vi "Add Subscriber.vi"(8 "error in (no error)":errorcluster, 10 "New FIFO Instance Config":T1, 11 "CIF_Fifo_Raw_Multi in":refnum<class "CIF_NIChn_Raw.lvclass">) -> (0 "error out":errorcluster, 2 "New Publisher":string, 3 "CIF_Fifo_Raw_Multi out":refnum<class "CIF_NIChn_Raw.lvclass">)   [LabVIEW 2021, in "CIF_NIChn_Raw.lvclass"]
uses:
  CIF_NIChn_Raw.lvclass
  D:/dev/Packages/Channel_Manager/src/CIFChannels/CIFChannels.lvclass
  D:/dev/Packages/Channel_Manager/src/CIF_NIChn/FIFO_U8_Multi/CIF_Fifo_U8_Multi.lvclass
  ChannelCommon/typedef/New FIFO Instance Configuration.ctl
  CIF_NIChn_Raw.lvclass/CIF_NIChn_Raw.ctl
  FIFO_U8_Multi/CIF_Fifo_U8_Multi.lvclass/CIF_Fifo_U8_Multi.ctl
  CIFChannels/Typedef/Direction.ctl
  FIFO_U8_Multi/Accessors/Read Publishers.vi
  FIFO_U8_Multi/Accessors/Write Publishers.vi
  FIFO_U8/CIF_NIChn_Fifo_U8.lvclass
  CIFChannels/CIFChannels.lvclass
  ChannelCommon/ChannelCommon.lvlib
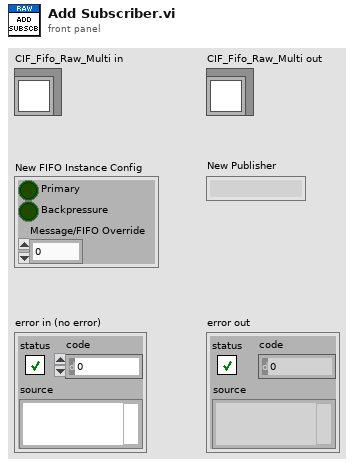
[diagram p1: front panel]
types:
  T1 = typedef "ChannelCommon.lvlib/New FIFO Instance Configuration.ctl" = cluster{"Primary":bool, "Backpressure":bool, "Message/FIFO Override":u32}
  T2 = typedef "CIFChannels.lvclass/Direction.ctl" = enum16{"Publisher", "Subscriber"}
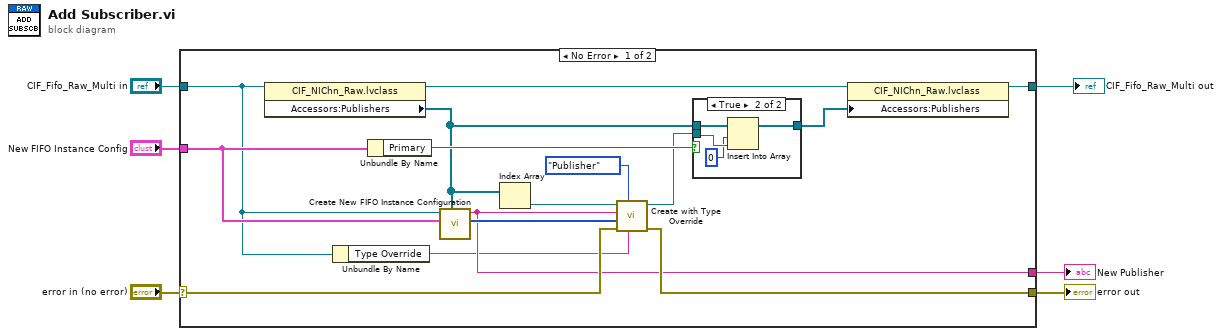
[diagram p0: block diagram]
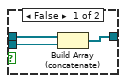
[diagram p2: hidden frame]
diagram:
  n1 = case shown="No Error" "error in (no error)" {
    selector: "error in (no error)" -> [w15 w30]
    tunnel: [w14 w30] -> w1
    tunnel: [w17 w29] -> w4
    tunnel: "CIF_Fifo_Raw_Multi in" -> [w8 w29]
    tunnel: "New FIFO Instance Config" -> [w20 _]
    tunnel: [w12 _] -> w6
    frame No Error {
      n2 = property class="CIF_NIChn_Raw.lvclass"(reference=w8) -> (reference out=w18:refnum<class "CIF_NIChn_Raw.lvclass">, "Accessors:Publishers"=w19:refnum<class "CIF_NIChn_Fifo_U8.lvclass">[])  [unwired: 1 in, 1 out]
      n3 = Unbundle By Name(w8) -> ("Type Override"=w7:string)
      n4 = Unbundle By Name(w20) -> ("Primary"=w21:bool)
      n5 = call "Create New FIFO Instance Configuration.vi"("Publisher Array in"=w19, "New FIFO Instance Config"=w20, "CIFChannels.lvclass"=w8) -> ("Flattened FIFO Config"=w13:u8[], "New Publisher"=w12:string)  [unwired: 7 in]
      n6 = Index Array(array=w19) -> (element=w10:refnum<class "CIF_NIChn_Fifo_U8.lvclass">)  [unwired: 1 in]
      n7 = call "Create with Type Override.vi"("Type Override"=w7, "Direction"=Direction."Publisher", "error in (no error)"=w15, "Custom Config Data"=w13, "Name"=w12, "CIFFIFO in"=w10) -> ("error out"=w14:errorcluster, "CIFFIFO out"=w9:refnum<class "CIF_NIChn_Fifo_U8.lvclass">)  [unwired: 4 in]
      n8 = case shown="True" w21 {
        tunnel: w19 -> [w24 w28]
        tunnel: [w23 w25] -> w16
        tunnel: w9 -> [w22 w27]
        frame False {
          n9 = Build Array (concatenate)(w24, w22) -> (w23:refnum<class "CIF_NIChn_Fifo_U8.lvclass">[])
        }
        frame True {
          n10 = Insert Into Array(array=w28, index=0, new element=w27) -> (w25:refnum<class "CIF_NIChn_Fifo_U8.lvclass">[])
        }
      }
      n11 = property class="CIF_NIChn_Raw.lvclass"(reference=w18, "Accessors:Publishers"=w16) -> (reference out=w17:refnum<class "CIF_NIChn_Raw.lvclass">)  [unwired: 1 in, 1 out]
    }
    frame Error {
    }
  }
  "error out" <- w1
  "CIF_Fifo_Raw_Multi out" <- w4
  "New Publisher" <- w6
